vi "DSF.Engine.Framework.Set Sequencer.vi"(10 "Sequencer":refnum<class "DSF.Engine.Sequencer.lvclass">, 11 "Framework in":refnum<class "DSF.Engine.Framework.lvclass">) -> (3 "Framework out":refnum<class "DSF.Engine.Framework.lvclass">)   [LabVIEW 2017, in "DSF.Engine.lvlib" / "DSF.Engine.Framework.lvclass"]
uses:
  DSF.Engine.Framework.lvclass
  Sequencer/DSF.Engine.Sequencer.lvclass
  DSF.Engine.Framework.lvclass/DSF.Engine.Framework.ctl
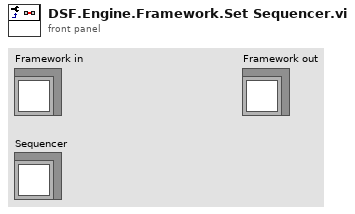
[diagram p1: front panel]
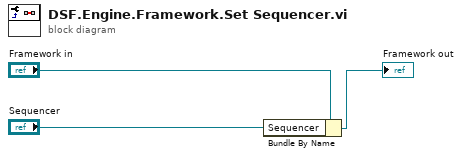
[diagram p0: block diagram]
diagram:
  n1 = Bundle By Name(cluster="Framework in", "Sequencer"="Sequencer") -> (→"Framework out":refnum<class "DSF.Engine.Framework.lvclass">)
